vi "SlitMoved.vi"(8 "error in (no error)":errorcluster, 9 "Slitwidth":u16, 10 "Slit":T1, 11 "SpectrometerComm in":refnum<class "SpectrometerComm.lvclass">) -> (0 "error out":errorcluster, 3 "SpectrometerComm out":refnum<class "SpectrometerComm.lvclass">)   [LabVIEW 2023, in "SpectrometerComm.lvclass"]
uses:
  SpectrometerComm.lvclass
  UIs/SinglePhoton_UI/typedefs/SpectrSlitControl.ctl
  typedefs/typedefs.lvlib
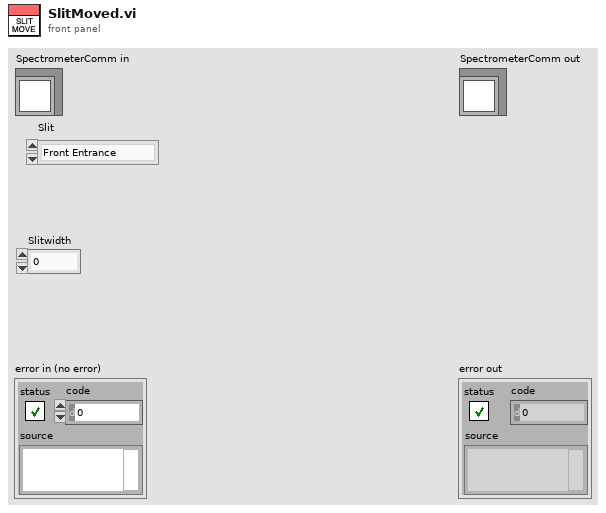
[diagram p1: front panel]
types:
  T1 = typedef "typedefs.lvlib/SpectrSlitControl.ctl" = enum16{"Front Entrance", "Side Entrance", "Front Exit", "Side Exit"}
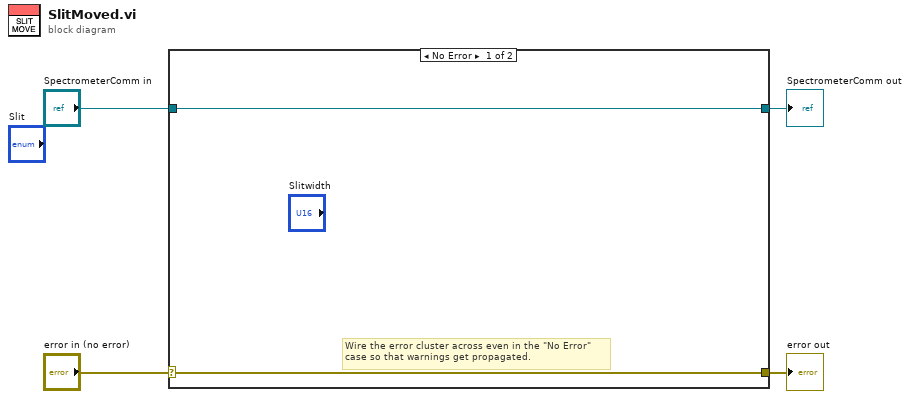
[diagram p0: block diagram]
diagram:
  n1 = case shown="No Error" "error in (no error)" {
    selector: "error in (no error)" -> [w5 w8]
    tunnel: [w5 w8] -> w3
    tunnel: [w6 w7] -> w1
    tunnel: "SpectrometerComm in" -> [w6 w7]
    frame No Error {
      # "Wire the error cluster across even in the \"No Error\"\ncase so that warnings get propagated."
    }
    frame Error {
    }
  }
  "error out" <- w3
  "SpectrometerComm out" <- w1
